vi "PH_Watchdog.constructor.vi"(0 "name":string, 2 "data in":string, 5 "error in(no error)":errorcluster) -> (14 "i ref out":refnum<vi>, 16 "data out":string, 19 "error out":errorcluster)   [LabVIEW 2014, in "PH_Watchdog.lvlib"]
doc: "This class is forseen to control black boxes (motion).\n\nThis class is part of the PHELIX device layer.\n\nauthor: Stefan Götte, GSI\n\nLicense Agreement for this software:\n\nCopyright (C)\nGesellschaft für Schwerionenforschung, GSI\nPlanckstr. 1\n64291 Darmstadt\nGermany\n\nContact: D.Beck@gsi.de \n\nThis program is free software; you can redistribute it and/or modify it under the terms of the \nGNU General Public License as published by the Free Software Foundation; either version 2 of \nthe license, or (at your option) any later version.\n\nThis program is distributed in the hope that it will be useful, but WITHOUT ANY WARRANTY; \nwithout even the implied warranty of MERCHANTABILITY or FITNESS FOR A PARTICULAR PURPOSE. See the GNU General License for more details (http://www.gnu.org).\n\nGesellschaft für Schwerionenforschung, GSI\nPlanckstr. 1, 64291 Darmstadt, Germany\nFor all questions and ideas contact: M.Richter@gsi.de, H.Brand@gsi.de or D.Beck@gsi.de.\nLast update: 16-JUN-2004"
uses:
  PH_Watchdog.lvlib
  CS_Core/CSObj/CSObj.lvlib
  PH_Basics/PH_Class/PH_Class.lvlib
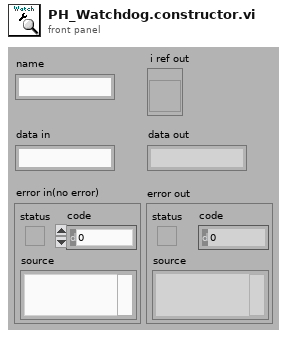
[diagram p1: front panel]
types:
  T1 = enum16{"SetAttribute", "GetAttribute", "CreateAttribute", "DestroyAttribute", "DestroyAllAtributes"}
  T2 = typedef "PH_Watchdog.lvlib/PH_Watchdog.i attribute.ctl" = cluster{"GUI Refs":cluster{"All":refnum<vi>, "Failures":refnum<vi>, "Alarms":refnum<vi>, "no info, but linked":refnum<vi>}, "All":T3[]}
  T3 = typedef "PH_Watchdog.lvlib/PH_Watchdog.Dataset.ctl" = cluster{"Instance":string, "Class":string, "Status":T4, "no Link":bool}
  T4 = typedef "PH_StatusHandler.lvlib/PH_StatusHandler.Status.ctl" = i16
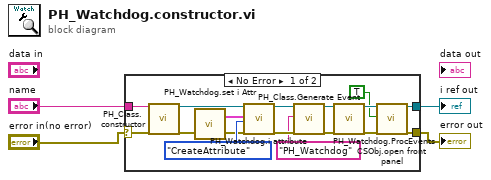
[diagram p0: block diagram]
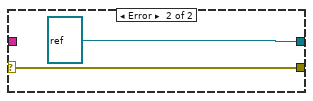
[diagram p2: hidden frame]
diagram:
  n1 = case shown="No Error" "error in(no error)" {
    selector: "error in(no error)" -> [w19 w23]
    tunnel: [w12 refnum<vi> refnum ("i ref out")] -> w4
    tunnel: [w14 w23] -> w3
    tunnel: "name" -> [w18 _]
    frame No Error {
      n2 = call "PH_Class.constructor.vi"("name"=w18, "error in"=w19) -> ("i ref out"=w20:refnum<vi>, "error out"=w7:errorcluster)  [unwired: 15 in, 1 out]
      n3 = call "PH_Watchdog.set i Attr.vi"("error in (no error)"=w7) -> ("error out"=w6:errorcluster, "i attribute"=w5:T2)  [unwired: 1 in]
      n4 = call "PH_Watchdog.i attribute.vi"("VI Refnum"=w20, "CLASS.i attribute"=w5, "Action"=T1."CreateAttribute", "error in (no error)"=w6) -> ("VI Refnum out"=w8:refnum<vi>, "error out"=w10:errorcluster)  [unwired: 13 in, 1 out]
      n5 = call "PH_Class.Generate Event.vi"("i ref in"=w8, "Class"="PH_Watchdog", "error in (no error)"=w10) -> ("i ref out"=w17:refnum<vi>, "error out"=w16:errorcluster)  [unwired: 15 in]
      n6 = call "PH_Watchdog.ProcEvents.vi"("i ref in"=w17, "error in (no error)"=w16) -> ("i ref out"=w13:refnum<vi>, "error out"=w15:errorcluster)  [unwired: 16 in]
      n7 = call "CSObj.open front panel.vi"("i ref in"=w13, "frontPanelOpen"=TRUE, "error in (no error)"=w15) -> ("i ref out"=w12:refnum<vi>, "error out"=w14:errorcluster)  [unwired: 15 in]
    }
    frame Error {
    }
  }
  "i ref out" <- w4
  "error out" <- w3
